vi "NanotecSMCPD.reset axis.vi"(0 "i ref in":refnum<vi>, 1 "axis":i32, 3 "ms timeout (10000)":i32=10000, 5 "error in (no error)":errorcluster) -> (14 "i ref out":refnum<vi>, 17 "timed out":bool, 19 "error out":errorcluster)   [LabVIEW 2014, in "NanotecSMCPD.lvlib"]
doc: "Resets the specified axis to the default values."
uses:
  NanotecSMCPD.lvlib
  CS_Core/CSSystem/CoreDefs/CoreDefs.error_type.ctl
  CS_Core/CSSystem/CoreDefs/CoreDefs.error_severity.ctl
  CSlibraries/UtilityLib/UtilityLib.valueStatus.ctl
  CS_Core/CSApplicationBaseClasses/DeviceBase/DeviceBase.lvlib
  CS_Core/CSSystem/CoreLib/CoreLib.lvlib
  CS_Core/CSApplicationBaseClasses/MotorBase/MotorBase.lvlib
  CSlibraries/UtilityLib/UtilityLib.lvlib
  instr.lib/NanotecSMCPD/NanotecSMCPDDriver.lvlib
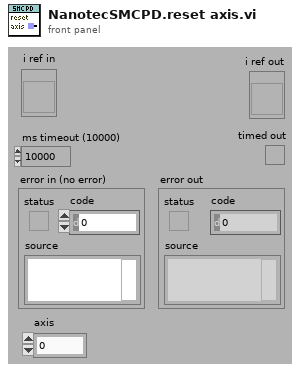
[diagram p1: front panel]
types:
  T1 = typedef "CoreDefs.error_severity.ctl" = enum16{"undefined", "information", "warning", "error", "fatal"}
  T2 = typedef "CoreDefs.error_type.ctl" = enum16{"no error", "can't load process", "can't unload process", "process does not exist", "can't install process", "can't remove process", "unknown function", "time out", "can't execute function", "duplicate queue name", "super not found", "caller queue invalid", "can't ping process", "unknown error", "VISA Error", "VISA timeout", "GPIB timeout", "GPIB error", "communication error", "data type mismatch", "can't read data from OPC server", "can't write data to OPC server", "OET error", "function not implemented", "process already exists", "invalid Shared Variable name", "error writing Shared Variable", "error reading Shared Variable", "invalid client name", "corrupt database", "unknown class", "call not authorized", "parameter out of range", "OET timeout: can't get data to modify", "invalid queue name", "requested operation incompatible with current state", "event undefined", "event disabled", "state undefined", "caller is not a friend", "EventBuilder: bad eventID", "EventBuilder: no DAQ devices", "a thread must not stop itself", "UNUSED ELEMENT4", "DiscArchiver: eventData incomplete", "DiscArchiver: eventData does not belong to run", "DiscArchiver: can't open file", "DiscArchiver: can't write to file", "DiscArchiver: available disc space low", "can't acquire semaphore", "error reading data from database", "notifier object is not existing", "can't register process", "can't unregister process", "illegal event type", "object disabled", "object already exists", "can't change state", "Instrument not found", "no connection to remote node", "invalid reference", "N/A", "UNUSED ELEMENT 1", "element not found", "illegal TCP/IP connection detected", "object does not exist", "invalid access ID", "unknown CS system", "invalid privilige", "unsupported data type", "unsupported server type", "IO server already exists", "Shared Variable already exists"}
  T3 = typedef "UtilityLib.lvlib/UtilityLib.valueStatus.ctl" = enum16{"no info available", "stand by/off", "on", "warning", "alarm/malfunction", "not implemented", "user action required", "important information", "system default", "control default", "indicator default", "button default"}
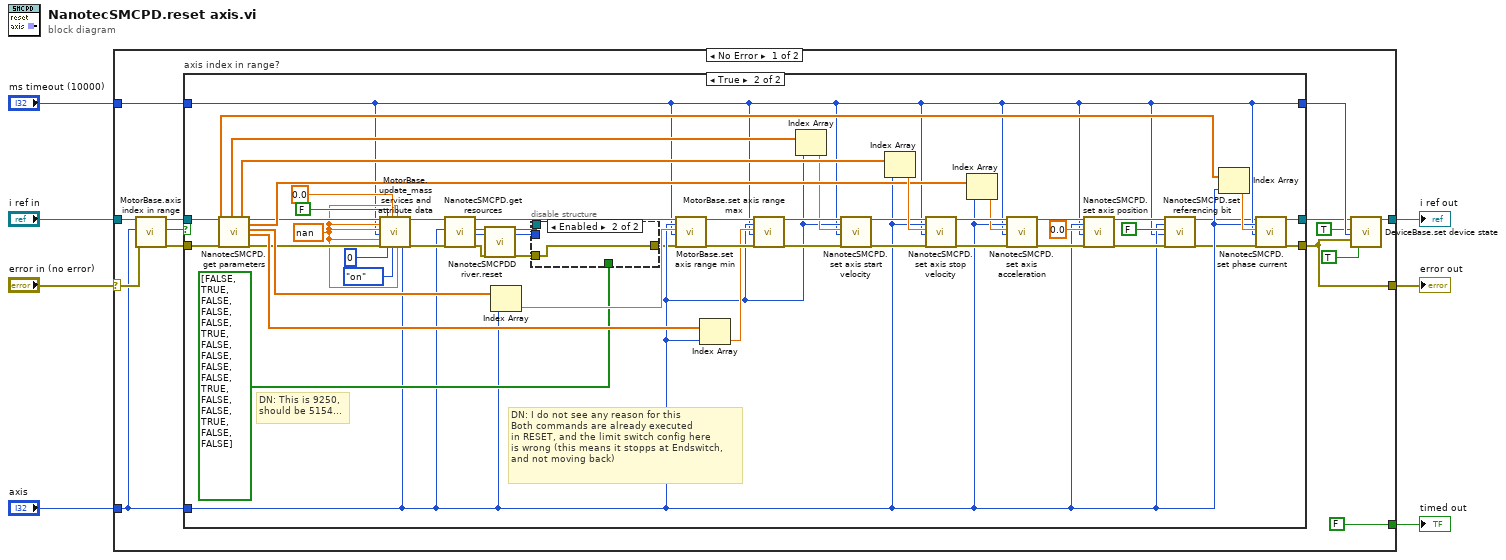
[diagram p0: block diagram]
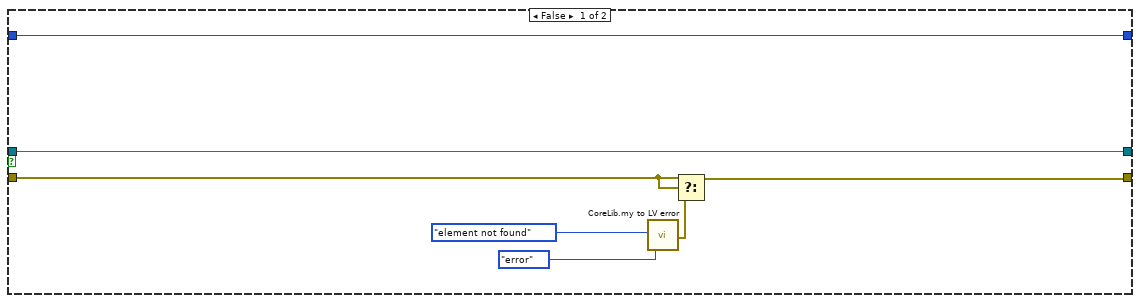
[diagram p2: hidden frame]
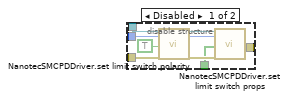
[diagram p3: hidden frame]
diagram:
  n1 = case shown="No Error" "error in (no error)" {
    selector: "error in (no error)" -> [w14 w90]
    tunnel: "ms timeout (10000)" -> [w11 _]
    tunnel: "i ref in" -> [w15 w91]
    tunnel: [w13 w90] -> w4
    tunnel: "axis" -> [w12 _]
    tunnel: [w10 w91] -> w2
    tunnel: [FALSE _] -> w1
    frame No Error {
      n2 = call "MotorBase.axis index in range.vi"("i ref in"=w15, "axisIndex"=w12, "error in (no error)"=w14) -> ("i ref out"=w19:refnum<vi>, "in range"=w18:bool, "error out"=w20:errorcluster)  [unwired: 14 in]
      n3 = case "axis index in range?" shown="True" w18 {
        tunnel: [w28 w37] -> w17
        tunnel: [w25 w38] -> w13
        tunnel: w11 -> [w22 w33]
        tunnel: w12 -> [_ w34]
        tunnel: w19 -> [w28 w80]
        tunnel: w20 -> [w26 w79]
        tunnel: [w22 w33] -> w21
        frame False {
          n4 = call "CoreLib.my to LV error.vi"("ErrorTypes"=CoreDefs.error_type."element not found", "severityLevel"=CoreDefs.error_severity."error") -> ("myErrorCluster"=w24:errorcluster)  [unwired: 16 in, 1 out]
          n5 = Select(t=w26, s=w26, f=w24) -> (s? t:f=w25:errorcluster)
        }
        frame True {
          w61 = nan ("startVelocity")
          # "DN: This is 9250, \nshould be 5154..."
          # "DN: I do not see any reason for this\nBoth commands are already executed\nin RESET, and the limit switch config here\nis wrong (this means it stopps at Endswitch,\nand not moving back)"
          n6 = call "NanotecSMCPD.get parameters.vi"("i ref in"=w80, "error in (no error)"=w79) -> ("startFrequency [unit/s]"=w76:dbl[], "PhaseCurrent [A]"=w35:dbl[], "stopFrequency [unit/s]"=w75:dbl[], "i ref out"=w69:refnum<vi>, "acceleration [unit/s^2]"=w71:dbl[], "minRange [unit]"=w78:dbl[], "maxRange[unit]"=w77:dbl[], "error out"=w66:errorcluster)  [unwired: 6 in, 4 out]
          n7 = call "MotorBase.update_mass services and attribute data.vi"("i ref in"=w69, "acceleration"=w61, "rangeMin"=w61, "ms timeout (10000)"=w33, "rangeMax"=w61, "error in (no error)"=w66, "onOff"=FALSE, "status"=0, "startVelocity"=0.0, "valueStatus"=UtilityLib.valueStatus."on", "stopVelocity"=w61, "position"=w61, "axisNumber"=w34) -> ("i ref out"=w68:refnum<vi>, "error out"=w67:errorcluster)  [unwired: 4 in, 1 out]
          n8 = call "NanotecSMCPD.get resources.vi"("i ref in"=w68, "axisNumber"=w34, "error in (no error)"=w67) -> ("i ref out"=w57:refnum<vi>, "VISA resource"=w52:refnum<visa-resource-name>, "address"=w51:i32, "error out"=w29:errorcluster)  [unwired: 13 in]
          n9 = call "NanotecSMCPDDriver.reset.vi"("VISA resource name"=w52, "contollerID"=w51, "error in (no error)"=w29) -> ("VISA resource name out"=w45:refnum<visa-resource-name>, "contollerID out"=w44:i32, "error out"=w43:errorcluster)  [unwired: 14 in]
          n10 = Index Array(array=w78, index=w34) -> (element=w56:dbl)
          n11 = disable-structure shown="Enabled" {
            disable-tunnel: w45 -> [w88 _]
            disable-tunnel: w44 -> [w87 _]
            disable-tunnel: w43 -> [w82 w89]
            disable-tunnel: bool[] [FALSE, TRUE, FALSE, FALSE, FALSE, TRUE, FALSE, FALSE, FALSE, FALSE, TRUE, FALSE, FALSE, TRUE, FALSE, FALSE] ("limitSwitchProperties (17442)") -> [w81 _]
            disable-tunnel: [_ w89] -> w30
            frame Disabled {
              n12 = call "NanotecSMCPDDriver.set limit switch polarity.vi"("VISA resource name"=w88, "contollerID"=w87, "normallyClosed"=TRUE, "error in (no error)"=w82) -> ("VISA resource name out"=w85:refnum<visa-resource-name>, "contollerID out"=w84:i32, "error out"=w83:errorcluster)  [unwired: 13 in]
              n13 = call "NanotecSMCPDDriver.set limit switch props.vi"("VISA resource name"=w85, "contollerID"=w84, "limitSwitchProperties (17442)"=w81, "error in (no error)"=w83) -> ()  [unwired: 13 in, 3 out]
            }
            frame Enabled {
            }
          }
          n14 = call "MotorBase.set axis range min.vi"("i ref in"=w57, "axis"=w34, "rangeMin [unit]"=w56, "ms timeout (10000)"=w33, "error in (no error)"=w30) -> ("i ref out"=w55:refnum<vi>, "error out"=w54:errorcluster)  [unwired: 12 in, 1 out]
          n15 = Index Array(array=w77, index=w34) -> (element=w53:dbl)
          n16 = call "MotorBase.set axis range max.vi"("i ref in"=w55, "axis"=w34, "rangeMax [unit]"=w53, "ms timeout (10000)"=w33, "error in (no error)"=w54) -> ("i ref out"=w50:refnum<vi>, "error out"=w48:errorcluster)  [unwired: 12 in, 1 out]
          n17 = Index Array(array=w76, index=w34) -> (element=w49:dbl)
          n18 = call "NanotecSMCPD.set axis start velocity.vi"("i ref in"=w50, "axis"=w34, "velocity [units/s]"=w49, "ms timeout (10000)"=w33, "error in (no error)"=w48) -> ("i ref out"=w47:refnum<vi>, "error out"=w46:errorcluster)  [unwired: 12 in, 1 out]
          n19 = Index Array(array=w75, index=w34) -> (element=w74:dbl)
          n20 = call "NanotecSMCPD.set axis stop velocity.vi"("i ref in"=w47, "axis"=w34, "velocity [units/s]"=w74, "ms timeout (10000)"=w33, "error in (no error)"=w46) -> ("i ref out"=w73:refnum<vi>, "error out"=w72:errorcluster)  [unwired: 12 in, 1 out]
          n21 = Index Array(array=w71, index=w34) -> (element=w70:dbl)
          n22 = call "NanotecSMCPD.set axis acceleration.vi"("i ref in"=w73, "axis"=w34, "acceleration [unit/s^2]"=w70, "ms timeout (10000)"=w33, "error in (no error)"=w72) -> ("i ref out"=w60:refnum<vi>, "error out"=w59:errorcluster)  [unwired: 12 in, 1 out]
          n23 = call "NanotecSMCPD.set axis position.vi"("i ref in"=w60, "axis"=w34, "position"=0.0, "ms timeout (10000)"=w33, "error in (no error)"=w59) -> ("i ref out"=w41:refnum<vi>, "error out"=w40:errorcluster)  [unwired: 12 in, 1 out]
          n24 = call "NanotecSMCPD.set referencing bit.vi"("i ref in"=w41, "axis"=w34, "isReferencing?"=FALSE ("referencing?"), "ms timeout (10000)"=w33, "error in (no error)"=w40) -> ("i ref out"=w31:refnum<vi>, "error out"=w32:errorcluster)  [unwired: 12 in, 1 out]
          n25 = Index Array(array=w35, index=w34) -> (element=w36:dbl)
          n26 = call "NanotecSMCPD.set phase current.vi"("i ref in"=w31, "axis"=w34, "phase current [A]"=w36, "ms timeout (10000)"=w33, "error in (no error)"=w32) -> ("i ref out"=w37:refnum<vi>, "error out"=w38:errorcluster)  [unwired: 12 in, 1 out]
        }
      }
      n27 = call "DeviceBase.set device state.vi"("i ref in"=w17, "implicit"=TRUE, "ms timeout (10000)"=w21, "device error"=w13, "mayResetError (FALSE)"=TRUE) -> ("i ref out"=w10:refnum<vi>)  [unwired: 12 in, 2 out]
    }
    frame Error {
    }
  }
  "error out" <- w4
  "i ref out" <- w2
  "timed out" <- w1
